vi "Booleans.vi"(7 "Array 2":T1(array[cluster])=[{"Boolean"=TRUE, "Radio Buttons"=enum."Radio Selection 2", "Boolean 2"=FALSE, "Array"=[TRUE, FALSE, FALSE, TRUE, FALSE, TRUE]}, {"Boolean"=FALSE, "Radio Buttons"=enum."Radio Selection 1", "Boolean 2"=TRUE, "Array"=[FALSE, FALSE, TRUE, FALSE, FALSE, TRUE]}], 8 "Array":bool[](array[boolean])=[FALSE, TRUE, FALSE, TRUE, FALSE, TRUE], 9 "Cluster":T2={"Boolean"=FALSE, "Radio Buttons"=enum."Radio Selection 1", "Boolean 2"=TRUE, "Array"=[TRUE, FALSE, TRUE, FALSE, TRUE]}, 10 "Boolean":bool) -> ()   [LabVIEW 2013]
panel:
  in  "stop":bool
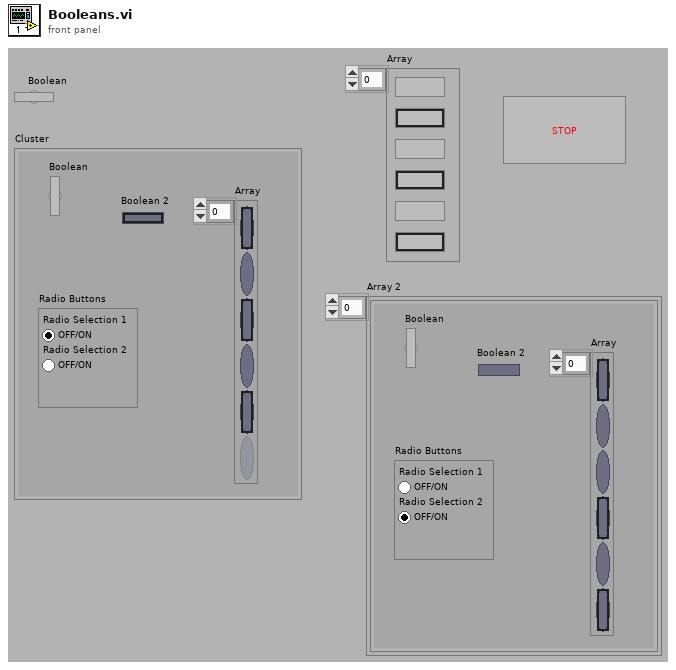
[diagram p1: front panel]
types:
  T1 = cluster{"Boolean":bool, "Radio Buttons":enum32{"Radio Selection 1", "Radio Selection 2"}, "Boolean 2":bool, "Array":bool[]}[]
  T2 = cluster{"Boolean":bool, "Radio Buttons":enum32{"Radio Selection 1", "Radio Selection 2"}, "Boolean 2":bool, "Array":bool[]}
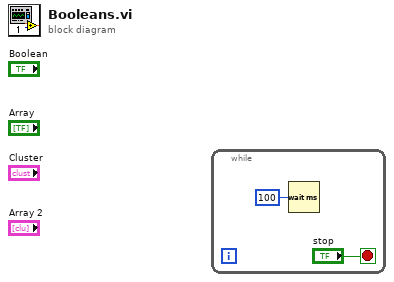
[diagram p0: block diagram]
diagram:
  n1 = while {
    stop <- "stop" stop-if-true
    n2 = Wait (ms)(milliseconds to wait=u32 100) -> ()  [unwired: 1 out]
  }
